vi "ExportDemos.vi"() -> ()   [LabVIEW 2013]
panel:
  in  "Output Dir":path
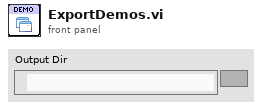
[diagram p1: front panel]
types:
  T1 = typedef "imagedata.ctl" = cluster{"image type":i32, "image depth":i32, "image":u8[], "mask":u8[], "colors":u32[], "Rectangle":cluster{"left":i16, "top":i16, "right":i16, "bottom":i16}}
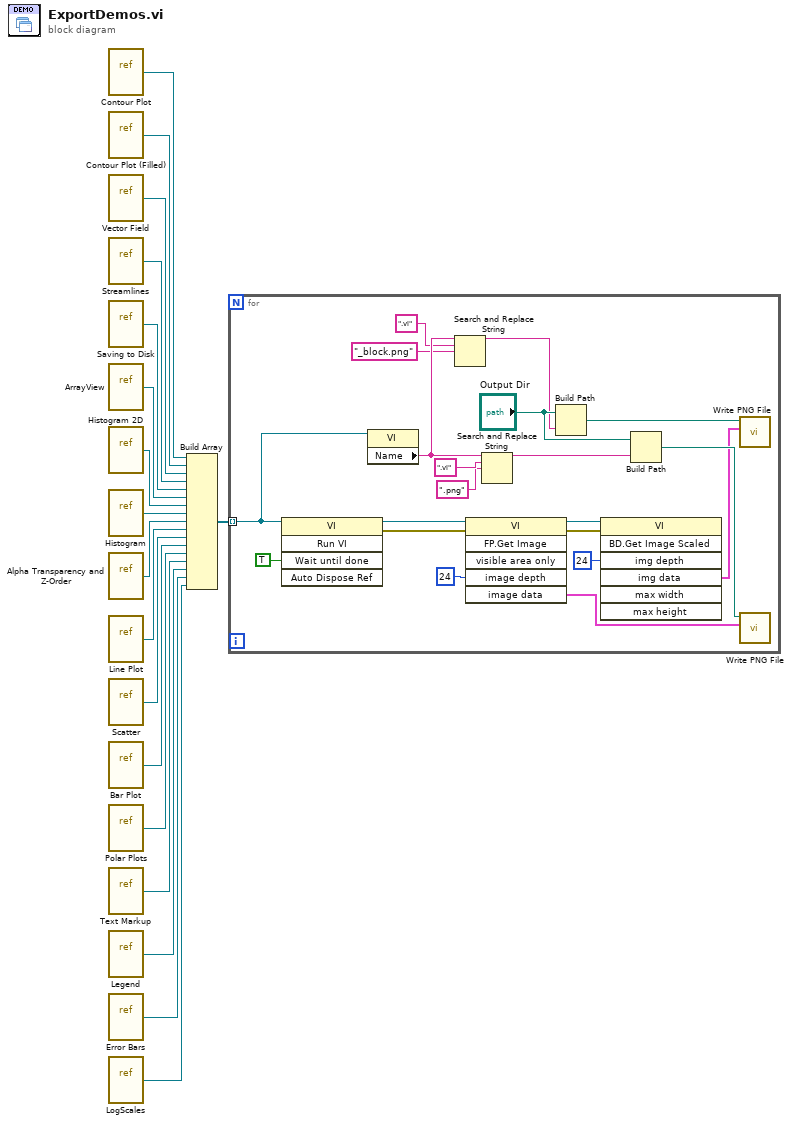
[diagram p0: block diagram]
diagram:
  n1 = vi-ref "Contour Plot.vi"() -> (w2:refnum<vi>)
  n2 = vi-ref "Contour Plot (Filled).vi"() -> (w18:refnum<vi>)
  n3 = vi-ref "Vector Field.vi"() -> (w17:refnum<vi>)
  n4 = vi-ref "Streamlines.vi"() -> (w16:refnum<vi>)
  n5 = vi-ref "Saving to Disk.vi"() -> (w3:refnum<vi>)
  n6 = vi-ref "ArrayView.vi"() -> (w15:refnum<vi>)
  n7 = vi-ref "Histogram 2D.vi"() -> (w14:refnum<vi>)
  n8 = vi-ref "Histogram.vi"() -> (w13:refnum<vi>)
  n9 = vi-ref "Alpha Transparency and Z-Order.vi"() -> (w12:refnum<vi>)
  n10 = vi-ref "Line Plot.vi"() -> (w11:refnum<vi>)
  n11 = vi-ref "Scatter.vi"() -> (w10:refnum<vi>)
  n12 = vi-ref "Bar Plot.vi"() -> (w9:refnum<vi>)
  n13 = vi-ref "Polar Plots.vi"() -> (w8:refnum<vi>)
  n14 = vi-ref "Text Markup.vi"() -> (w7:refnum<vi>)
  n15 = vi-ref "Legend.vi"() -> (w6:refnum<vi>)
  n16 = vi-ref "Error Bars.vi"() -> (w5:refnum<vi>)
  n17 = vi-ref "LogScales.vi"() -> (w4:refnum<vi>)
  n18 = Build Array(w2, w18, w17, w16, w3, w15, w14, w13, w12, w11, w10, w9, w8, w7, w6, w5, w4) -> (w1:refnum<vi>[])
  n19 = for {
    tunnel: w1 -> [w20] mode=indexing
    n20 = invoke class="VI" method="Run VI"(reference=w20, "Wait until done"=TRUE ("Wait Until Done")) -> (reference out=w31:refnum<vi>, error out=w22:errorcluster)  [unwired: 3 in, 3 out]
    n21 = property class="VI"(reference=w20) -> ("Name"=w29:string)  [unwired: 1 in, 2 out]
    n22 = Search and Replace String(input string=w29, search string=".vi", replace string="_block.png" ("replace string (\"\")")) -> (result string=w24:string)  [unwired: 5 in, 3 out]
    n23 = invoke class="VI" method="FP.Get Image"(reference=w31, error in=w22, "image depth"=24 ("Image Depth")) -> (reference out=w30:refnum<vi>, error out=w21:errorcluster, "image data"=w38:T1)  [unwired: 3 in, 3 out]
    n24 = Search and Replace String(input string=w29, search string=".vi", replace string=".png" ("replace string (\"\")")) -> (result string=w34:string)  [unwired: 5 in, 3 out]
    n25 = Build Path(base path="Output Dir", name or relative path=w24) -> (appended path=w26:path)
    n26 = invoke class="VI" method="BD.Get Image Scaled"(reference=w30, error in=w21, "img depth"=24 ("Image Depth")) -> ("img data"=w23:T1)  [unwired: 4 in, 6 out]
    n27 = Build Path(base path="Output Dir", name or relative path=w34) -> (appended path=w37:path)
    n28 = call <vilib>:"Write PNG File.vi"("image data"=w23, "path to PNG file"=w26) -> ()  [unwired: 8 in, 2 out]
    n29 = call <vilib>:"Write PNG File.vi"("image data"=w38, "path to PNG file"=w37) -> ()  [unwired: 8 in, 2 out]
  }
